vi "Get_Circ_Area.vi"(4 "Radius":dbl) -> (1 "Area":dbl)   [LabVIEW 2011]
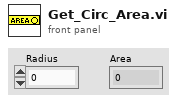
[diagram p1: front panel]
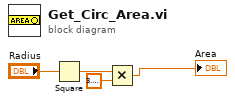
[diagram p0: block diagram]
diagram:
  n1 = Square(x="Radius") -> (x^2=w2:dbl)
  n2 = Multiply(x=w2, y=3.141592653589793) -> (x*y=→"Area":dbl)
